vi "test_Remove Waveform Input Channels.vi"(8 "error in (no error)":errorcluster, 11 "TestCase in":refnum<class "FPGA Addon Adding a Channel Item.lvclass">) -> (0 "error out":errorcluster, 3 "TestCase out":refnum<class "FPGA Addon Adding a Channel Item.lvclass">)   [LabVIEW 2019, in "FPGA Addon Adding a Channel Item.lvclass"]
uses:
  FPGA Addon Adding a Channel Item.lvclass
  Addon/Addon Shared/Types/FG Action.ctl
  FPGA Addon Adding a Channel Item.lvclass/FPGA Addon Adding a Channel Item.ctl
  Addon/Addon Shared/SubVIs/Constants.vi
  <vilib>/NI VeriStand/Custom Device Tools/Custom Device Utility Library/NI VeriStand - Search for Item by GUID.vi
  <vilib>/NI/NI VeriStand Advanced SysDef API/SysDef API/SysDef.Property.Get.vi
  <vilib>/NI/NI VeriStand Advanced SysDef API/_SubVIs/SysDef.Property.Get.Variant.vi
  <vilib>/NI/NI VeriStand Advanced SysDef API/SysDef API/SysDef.Property.Set.vi
  <vilib>/NI/NI VeriStand Advanced SysDef API/_SubVIs/SysDef.Property.Set.Variant.vi
  <vilib>/NI/NI VeriStand Advanced SysDef API/_SubVIs/SysDef.Search.GUIDs.vi
  <vilib>/addons/_JKI Toolkits/VI Tester/TestCase.llb/TestCase.lvclass
  Addon/Addon System Explorer/FPGA Addon System Explorer.lvlib
  Addon/Addon Shared/FPGA Addon Shared.lvlib
  <vilib>/NI VeriStand/Custom Device Tools/Custom Device Utility Library/Custom Device Utility Library.lvlib
  <vilib>/NI/NI VeriStand Advanced SysDef API/SysDef API/Advanced System Definition.lvlib
  C:/Program Files (x86)/National Instruments/LabVIEW 2019/vi.lib/addons/_JKI Toolkits/VI Tester/TestCase.llb/TestCase.lvclass
panel:
  out "GUIDs":string[](array[string])
  in  "remove":bool
  in  "add":bool
  out "Names":string[](array[string])
  in  "Available Registers":i32[](listbox)
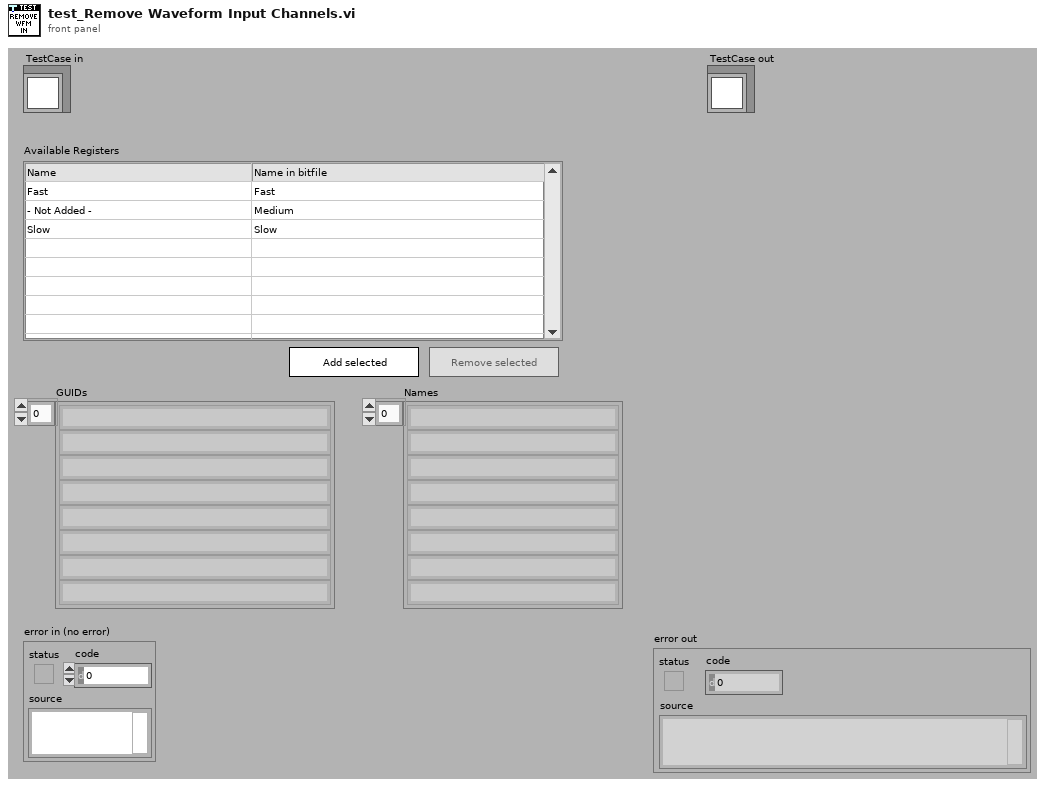
[diagram p1: front panel]
types:
  T1 = typedef "FPGA Addon Shared.lvlib/FG Action.ctl" = enum8{"GET", "SET"}
  T2 = typedef "Custom Device API.lvlib/Custom Device Item Ref.ctl" = u64
  T3 = typedef "FPGA Addon Shared.lvlib/DMA Information.ctl" = cluster{"Name":string, "Data Type":T4}
  T4 = typedef "FPGA Addon Shared.lvlib/Data Type.ctl" = enum8{"<Null>", "I8", "I16", "I32", "I64", "U8", "U16", "U32", "U64", "SGL", "Boolean", "Analog PWM In Settings", "Analog PWM In", "Digital PWM In Settings", "Digital PWM In", "Digital PWM Out", "Sine Out", "FXP+/-24.5", "FXP+/-16.5", "FXP+/-32.8", "FXP+/-64.32", "FXP+/-16.7", "FXP+/-20.5", "FXP+/-27.5", "FXP+/-32.16", "FXP+16.3", "FXP+18.3", "Digital Static In", "Digital Static Out", "Digital Static In Settings", "Digital WSS Out", "Quad Encoder Settings", "Quad Encoder In", "Group"}
  T5 = typedef "FPGA Addon System Explorer.lvlib/Listbox Cluster.ctl" = cluster{"add":refnum<vi>, "remove":refnum<vi>, "Listbox":refnum<vi>, "selected":i32[], "not present":i32[], "listbox text":string[][], "Section Ref":T2}
  T6 = typedef "Advanced System Definition.lvlib/TreeItem.Info.ctl" = cluster{"Name":string, "Description":string, "GUID":string, "Is Channel":bool, "Channel":T7, "Is Waveform":bool, "Waveform":T9}
  T7 = typedef "Custom Device API.lvlib/Custom Device Channel.ctl" = cluster{"Type":T8, "Units":string, "Default Value":dbl, "Faultable":bool, "Scalable":bool}
  T8 = typedef "Custom Device API.lvlib/Custom Device Channel Type.ctl" = enum16{"Input", "Output"}
  T9 = typedef "Custom Device API.lvlib/Custom Device Waveform.ctl" = cluster{"Data Type":T10, "Units":string}
  T10 = typedef "Custom Device API.lvlib/Custom Device Waveform DataType.ctl" = enum16{"Double", "Complex Double"}
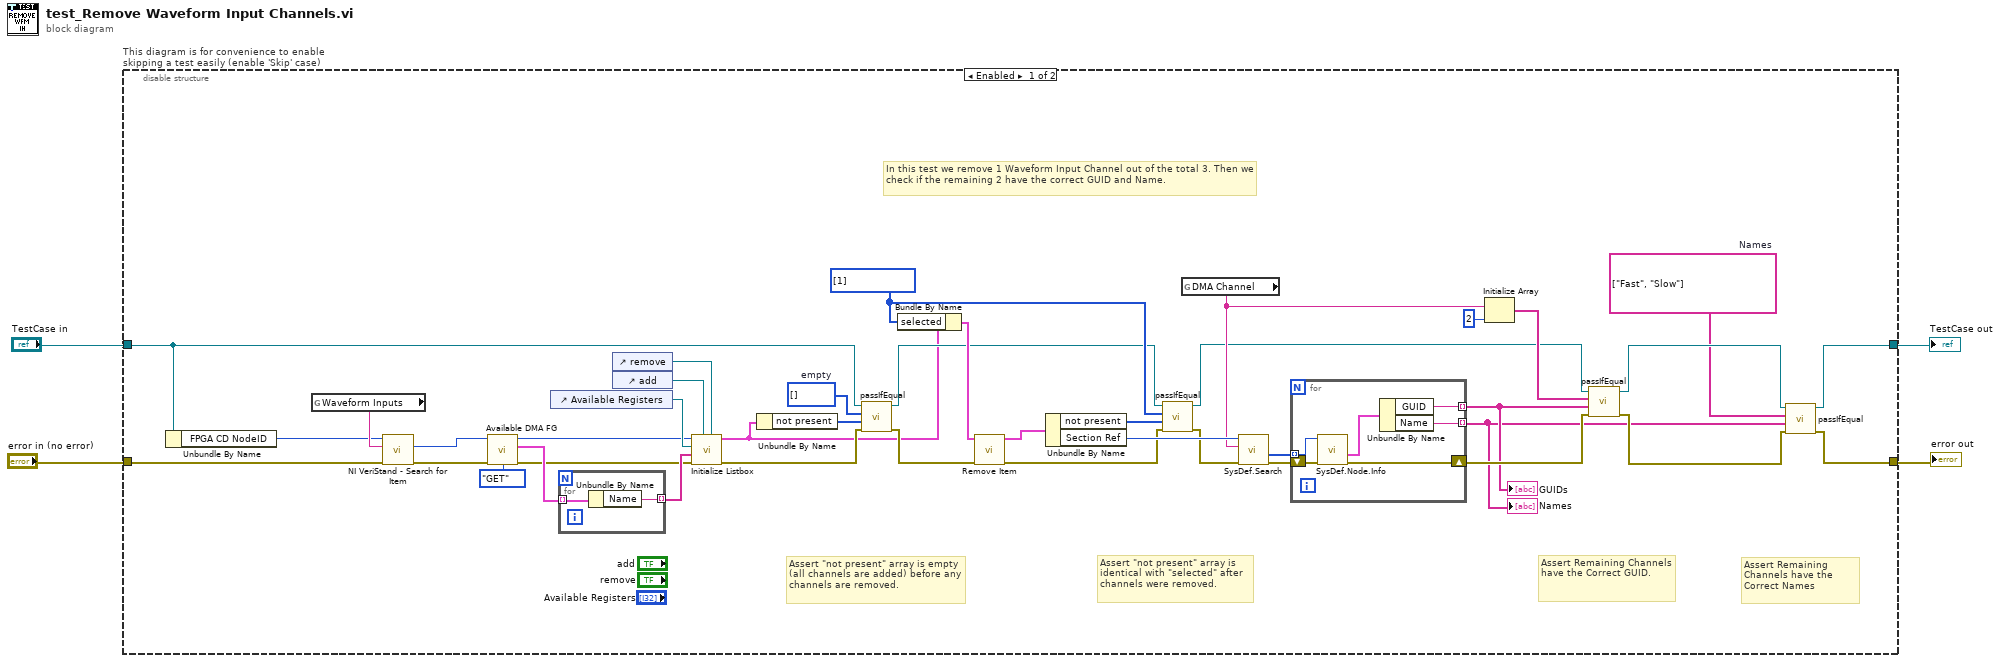
[diagram p0: block diagram]
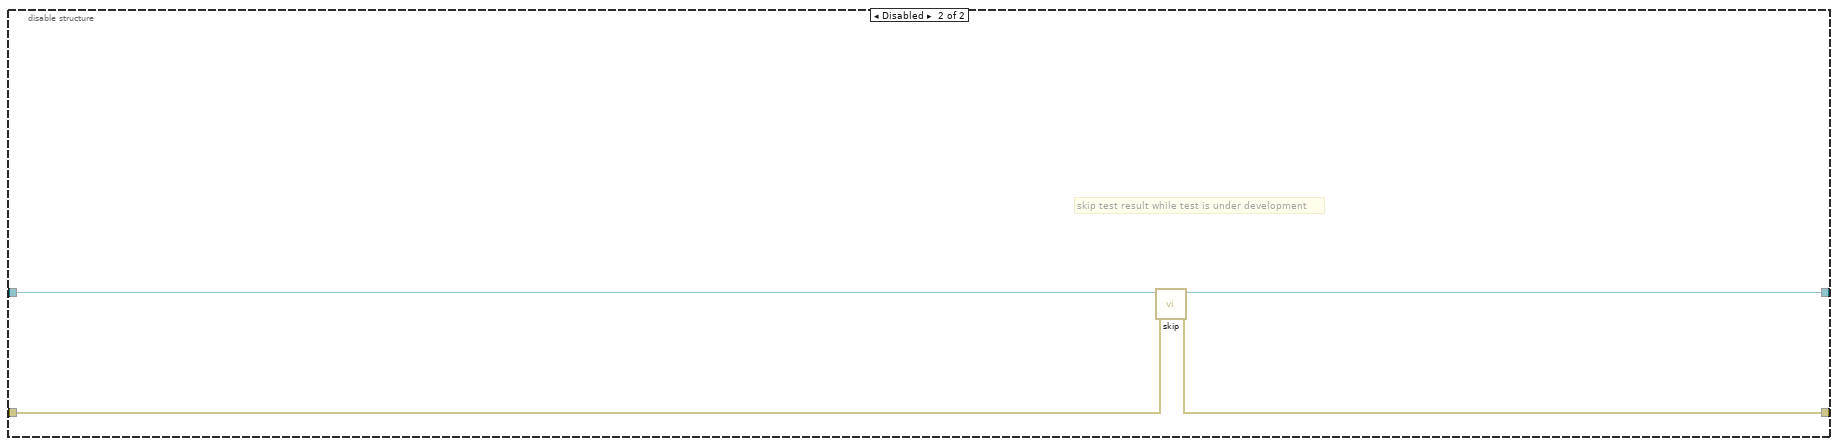
[diagram p2: hidden frame]
diagram:
  n1 = disable-structure "This diagram is for convenience to enable skipping a test easily (enable 'Skip' case)" shown="Enabled" {
    disable-tunnel: "TestCase in" -> [w9 w57]
    disable-tunnel: [w31 w55] -> w1
    disable-tunnel: [w30 w56] -> w3
    disable-tunnel: "error in (no error)" -> [w29 w54]
    frame Enabled {
      w10 = i32[] []  # empty
      w32 = string[] ["Fast", "Slow"]  # Names
      w18 = i32[] [1] ("selected")
      # "Assert \"not present\" array is empty (all channels are added) before any channels are removed."
      # "Assert \"not present\" array is identical with \"selected\" after channels were removed."
      # "In this test we remove 1 Waveform Input Channel out of the total 3. Then we check if the remaining 2 have the correct GUID and Name."
      # "Assert Remaining Channels have the Correct Names"
      # "Assert Remaining Channels have the Correct GUID."
      n2 = Unbundle By Name(w9) -> ("FPGA CD NodeID"=w28:u64)
      n3 = global read "Constants.vi" "Waveform Inputs"() -> (w43:string)
      n4 = call-poly <vilib>:"NI VeriStand - Search for Item.vi"("error in"=w29, "Item GUID"=w43, "Section Ref in"=w28) -> ("error out"=w16:errorcluster, "Item Ref"=w17:T2)  [unwired: 5 in, 2 out]
      n5 = call "Available DMA FG.vi"("Action"=FG_Action."GET", "error in (no error)"=w16, "Item Ref"=w17) -> ("error out"=w12:errorcluster, "Available DMA"=w13:T3[], "Item Ref out"=w14:T2)  [unwired: 6 in]
      n6 = control-ref of="Available Registers"() -> (w45:refnum<vi>)
      n7 = for {
        tunnel: w13 -> [w47] mode=indexing
        tunnel: [w46] -> w44 mode=indexing
        n8 = Unbundle By Name(w47) -> ("Name"=w46:string)
      }
      n9 = control-ref of="remove"() -> (w39:refnum<vi>)
      n10 = control-ref of="add"() -> (w40:refnum<vi>)
      n11 = call "Initialize Listbox.vi"("remove"=w39, "add"=w40, "error in (no error)"=w12, "Names"=w44, "Listbox"=w45, "Item Ref"=w14) -> ("error out"=w7:errorcluster, "Listbox Refs"=w5:T5)  [unwired: 4 in]
      n12 = Unbundle By Name(w5) -> ("not present"=w11:i32[])
      n13 = call-dynamic "passIfEqual.vi"("error in (no error)"=w7, "y"=w11, "x"=w10, "TestCase in"=w9) -> ("error out"=w6:errorcluster, "TestCase out"=w8:refnum<class "FPGA Addon Adding a Channel Item.lvclass">)  [unwired: 6 in]
      n14 = Bundle By Name(cluster=w5, "selected"=w18) -> (w25:T5)
      n15 = call "Remove Item.vi"("error in (no error)"=w6, "Listbox Refs in"=w25) -> ("error out"=w22:errorcluster, "Listbox Refs out"=w24:T5)  [unwired: 8 in]
      n16 = Unbundle By Name(w24) -> ("not present"=w20:i32[], "Section Ref"=w41:T2)
      n17 = call-dynamic "passIfEqual.vi"("error in (no error)"=w22, "y"=w20, "x"=w18, "TestCase in"=w8) -> ("error out"=w21:errorcluster, "TestCase out"=w19:refnum<class "FPGA Addon Adding a Channel Item.lvclass">)  [unwired: 6 in]
      n18 = global read "Constants.vi" "DMA Channel"() -> (w26:string)
      n19 = call-poly <vilib>:"SysDef.Search.vi"("error in (no error)"=w21, "GUID"=w26, "nodeID"=w41) -> ("error out"=w42:errorcluster, "Values Out"=w38:u64[])  [unwired: 5 in, 2 out]
      n20 = for {
        tunnel: w38 -> [w50] mode=indexing
        tunnel: [w48] -> w33 mode=indexing
        tunnel: [w49] -> w35 mode=indexing
        shift-right: [w52] -> w36
        shift-left: w42 -> [w53]
        n21 = call <vilib>:"SysDef.Node.Info.vi"("error in (no error)"=w53, "nodeID"=w50) -> ("error out"=w52:errorcluster, "Item Info"=w51:T6)  [unwired: 6 in, 2 out]
        n22 = Unbundle By Name(w51) -> ("GUID"=w49:string, "Name"=w48:string)
      }
      "Names" <- w33
      "GUIDs" <- w35
      n23 = Initialize Array(w26, 2 ("dimension size")) -> (w27:string[])
      n24 = call-dynamic "passIfEqual.vi"("error in (no error)"=w36, "y"=w35, "x"=w27, "TestCase in"=w19) -> ("error out"=w37:errorcluster, "TestCase out"=w34:refnum<class "FPGA Addon Adding a Channel Item.lvclass">)  [unwired: 6 in]
      n25 = call-dynamic "passIfEqual.vi"("error in (no error)"=w37, "y"=w33, "x"=w32, "TestCase in"=w34) -> ("error out"=w30:errorcluster, "TestCase out"=w31:refnum<class "FPGA Addon Adding a Channel Item.lvclass">)  [unwired: 6 in]
    }
    frame Disabled {
      # "skip test result while test is under development"
      n26 = call <vilib>:"skip.vi"("error in (no error)"=w54, "TestCase in"=w57) -> ("error out"=w56:errorcluster, "TestCase out"=w55:refnum<class "FPGA Addon Adding a Channel Item.lvclass">)  [unwired: 8 in]
    }
  }
  "error out" <- w3
  "TestCase out" <- w1
